vi "Get Color.vi"(11 "Generic Plugin in":refnum<class "Generic Plugin.lvclass">) -> (3 "Color Box":u32(colorbox))   [LabVIEW 2019, in "Generic Plugin.lvclass"]
uses:
  Generic Plugin.lvclass
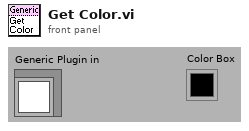
[diagram p1: front panel]
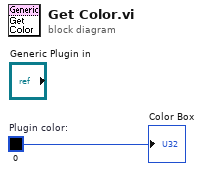
[diagram p0: block diagram]
diagram:
  w1 = u32 0  # Plugin color:
  "Color Box" <- w1
